vi "Main_09a refactored.vi"() -> ()   [LabVIEW 2020]
uses:
  Cluster_Point.ctl
panel:
  out "Tail Track":set{T1}(c389)
  in  "Puzzle Description":string="--- Day 9: Rope Bridge ---\nThis rope bridge creaks as you walk along it. You aren't sure how old it is, or whether it can even support your weight.\n\nIt seems to support the Elves just fine, though. The bridge spans a gorge which was carved out by the massive river far below you.\n\nYou step carefully; as you do, the ropes stretch and twist. You decide to distract yourself by modeling rope physics; maybe you can even figure out where not to step.\n\nConsider a rope with a knot at each end; these knots mark the head and the tail of the rope. If the head moves far enough away from the tail, the tail is pulled toward the head.\n\nDue to nebulous reasoning involving Planck lengths, you should be able to model the positions of the knots on a two-dimensional grid. Then, by following a hypothetical series of motions (your puzzle input) for the head, you can determine how the tail will move.\n\nDue to the aforementioned Planck lengths, the rope must be quite short; in fact, the head (H) and tail (T) must always be touching (diagonally adjacent and even overlapping both count as touching):\n\n....\n.TH.\n....\n\n....\n.H..\n..T.\n....\n\n...\n.H. (H covers T)\n...\nIf the head is ever two steps directly up, down, left, or right from the tail, the tail must also move one step in that direction so it remains close enough:\n\n.....    .....    .....\n.TH.. -> .T.H. -> ..TH.\n.....    .....    .....\n\n...    ...    ...\n.T.    .T.    ...\n.H. -> ... -> .T.\n...    .H.    .H.\n...    ...    ...\nOtherwise, if the head and tail aren't touching and aren't in the same row or column, the tail always moves one step diagonally to keep up:\n\n.....    .....    .....\n.....    ..H..    ..H..\n..H.. -> ..... -> ..T..\n.T...    .T...    .....\n.....    .....    .....\n\n.....    .....    .....\n.....    .....    .....\n..H.. -> ...H. -> ..TH.\n.T...    .T...    .....\n.....    .....    .....\nYou just need to work out where the tail goes as the head follows a series of motions. Assume the head and the tail both start at the same position, overlapping.\n\nFor example:\n\nR 4\nU 4\nL 3\nD 1\nR 4\nD 1\nL 5\nR 2\nThis series of motions moves the head right four steps, then up four steps, then left three steps, then down one step, and so on. After each step, you'll need to update the position of the tail if the step means the head is no longer adjacent to the tail. Visually, these motions occur as follows (s marks the starting position as a reference point):\n\n== Initial State ==\n\n......\n......\n......\n......\nH.....  (H covers T, s)\n\n== R 4 ==\n\n......\n......\n......\n......\nTH....  (T covers s)\n\n......\n......\n......\n......\nsTH...\n\n......\n......\n......\n......\ns.TH..\n\n......\n......\n......\n......\ns..TH.\n\n== U 4 ==\n\n......\n......\n......\n....H.\ns..T..\n\n......\n......\n....H.\n....T.\ns.....\n\n......\n....H.\n....T.\n......\ns.....\n\n....H.\n....T.\n......\n......\ns.....\n\n== L 3 ==\n\n...H..\n....T.\n......\n......\ns.....\n\n..HT..\n......\n......\n......\ns.....\n\n.HT...\n......\n......\n......\ns.....\n\n== D 1 ==\n\n..T...\n.H....\n......\n......\ns.....\n\n== R 4 ==\n\n..T...\n..H...\n......\n......\ns.....\n\n..T...\n...H..\n......\n......\ns.....\n\n......\n...TH.\n......\n......\ns.....\n\n......\n....TH\n......\n......\ns.....\n\n== D 1 ==\n\n......\n....T.\n.....H\n......\ns.....\n\n== L 5 ==\n\n......\n....T.\n....H.\n......\ns.....\n\n......\n....T.\n...H..\n......\ns.....\n\n......\n......\n..HT..\n......\ns.....\n\n......\n......\n.HT...\n......\ns.....\n\n......\n......\nHT....\n......\ns.....\n\n== R 2 ==\n\n......\n......\n.H....  (H covers T)\n......\ns.....\n\n......\n......\n.TH...\n......\ns.....\nAfter simulating the rope, you can count up all of the positions the tail visited at least once. In this diagram, s again marks the starting position (which the tail also visited) and # marks other positions the tail visited:\n\n..##..\n...##.\n.####.\n....#.\ns###..\nSo, there are 13 positions the tail visited at least once.\n\nSimulate your complete hypothetical series of motions. How many positions does the tail of the rope visit at least once?"
  out "Tail Positon count":i32
  in  "Puzzle":string="R 1\nD 1\nL 1\nD 1\nR 2\nL 1\nU 2\nD 1\nU 2\nL 1\nU 1\nL 2\nD 1\nU 2\nL 1\nR 1\nD 1\nL 2\nD 2\nL 2\nR 1\nL 2\nU 2\nR 2\nL 2\nU 2\nL 1\nD 1\nL 2\nU 1\nR 1\nD 2\nL 2\nU 1\nR 1\nD 1\nU 2\nL 1\nD 2\nU 1\nD 1\nR 2\nD 1\nL 2\nD 1\nL 1\nR 1\nD 2\nL 1\nR 2\nD 2\nU 2\nR 2\nD 2\nR 2\nL 2\nD 2\nL 2\nD 1\nU 2\nR 1\nD 2\nL 2\nR 2\nL 1\nD 1\nU 2\nD 1\nR 2\nU 2\nR 2\nD 1\nL 1\nU 2\nD 1\nU 1\nD 2\nU 1\nR 1\nU 2\nD 1\nL 2\nU 1\nL 2\nD 2\nR 1\nU 2\nL 1\nD 2\nR 1\nU 1\nD 1\nL 2\nU 1\nR 1\nD 2\nU 2\nL 1\nU 2\nD 2\nR 1\nU 2\nR 1\nU 2\nR 1\nD 2\nU 1\nD 2\nL 2\nD 2\nL 2\nD 2\nR 1\nU 1\nD 3\nU 1\nR 2\nU 3\nD 1\nU 2\nD 2\nU 2\nD 1\nU 2\nR 2\nL 2\nU 1\nL 3\nD 1\nR 3\nD 3\nR 2\nL 1\nU 3\nD 1\nU 2\nR 2\nD 1\nR 3\nD 2\nR 3\nD 1\nU 3\nL 3\nR 2\nU 3\nL 3\nU 2\nL 3\nD 1\nR 3\nU 3\nR 2\nD 1\nU 3\nR 3\nD 1\nL 2\nD 2\nL 2\nD 3\nR 2\nU 3\nL 3\nD 2\nU 3\nL 2\nU 3\nD 1\nL 1\nD 3\nR 1\nD 3\nU 1\nL 3\nU 1\nD 2\nU 1\nD 1\nU 2\nD 3\nL 1\nU 1\nR 1\nU 3\nD 3\nR 1\nL 2\nR 3\nL 3\nU 1\nD 2\nR 2\nU 2\nD 3\nU 2\nD 3\nL 1\nR 3\nD 3\nR 2\nU 3\nD 3\nL 2\nR 3\nD 3\nR 2\nL 1\nR 3\nD 2\nR 1\nD 3\nL 1\nU 1\nD 2\nR 1\nD 1\nL 1\nR 2\nL 1\nU 1\nL 2\nD 2\nL 2\nD 1\nL 2\nU 3\nD 1\nR 3\nL 2\nR 1\nL 2\nR 3\nU 2\nL 4\nR 3\nL 1\nR 2\nD 2\nL 4\nU 3\nL 1\nD 1\nL 3\nU 2\nL 3\nU 2\nL 1\nR 2\nL 3\nU 1\nD 2\nR 1\nL 4\nR 4\nL 4\nU 2\nD 2\nR 2\nL 2\nU 2\nR 1\nD 3\nL 4\nR 2\nU 1\nL 4\nR 1\nL 1\nD 4\nR 3\nD 1\nR 2\nL 2\nR 3\nL 1\nU 1\nD 3\nU 2\nR 1\nL 1\nD 3\nR 2\nU 2\nR 3\nU 2\nD 1\nR 4\nU 4\nD 3\nU 3\nR 2\nU 1\nL 1\nU 4\nD 1\nR 4\nD 4\nL 3\nU 4\nR 4\nL 1\nR 1\nU 2\nR 4\nD 2\nR 1\nU 2\nL 1\nD 1\nL 3\nR 3\nL 3\nD 3\nL 4\nD 2\nU 2\nD 3\nR 1\nU 1\nD 3\nU 1\nR 3\nD 2\nL 3\nR 2\nD 1\nL 3\nD 3\nU 3\nD 4\nL 2\nU 3\nD 5\nL 2\nD 2\nR 2\nL 3\nD 5\nU 4\nR 1\nD 5\nR 1\nD 1\nL 2\nR 4\nU 2\nD 3\nR 5\nL 2\nR 2\nD 1\nR 2\nU 5\nL 4\nU 5\nD 1\nL 2\nU 2\nR 2\nD 4\nU 3\nL 2\nD 1\nU 4\nL 4\nD 3\nL 3\nD 3\nR 1\nU 1\nR 1\nU 1\nR 2\nD 3\nR 5\nU 1\nD 2\nL 5\nU 5\nL 4\nD 4\nU 4\nL 1\nR 5\nU 2\nL 3\nU 2\nD 3\nL 5\nD 5\nL 2\nU 2\nD 4\nU 3\nD 3\nL 1\nD 2\nR 2\nD 1\nR 4\nL 3\nD 1\nU 4\nL 1\nR 2\nL 4\nD 5\nR 3\nD 1\nL 5\nD 5\nU 3\nR 2\nD 4\nL 2\nR 2\nD 3\nR 3\nU 2\nR 5\nU 4\nR 3\nL 1\nD 2\nU 1\nL 1\nR 2\nU 4\nD 4\nL 1\nR 1\nU 4\nL 3\nU 5\nR 3\nL 4\nD 3\nU 1\nR 4\nU 1\nL 1\nU 3\nR 4\nL 5\nD 1\nU 4\nR 5\nL 1\nR 4\nD 2\nL 6\nD 5\nU 5\nL 5\nR 6\nD 1\nU 2\nR 1\nU 4\nD 6\nL 6\nD 6\nU 6\nD 4\nU 4\nD 1\nU 3\nL 5\nD 6\nR 1\nL 1\nD 2\nL 4\nD 4\nL 4\nR 4\nU 2\nL 3\nD 4\nR 3\nD 4\nU 5\nR 4\nU 1\nR 6\nL 3\nR 2\nU 1\nL 1\nR 2\nD 3\nR 6\nD 6\nU 1\nD 3\nU 4\nD 5\nL 5\nU 3\nD 6\nL 5\nR 5\nU 1\nR 4\nD 2\nL 2\nR 4\nL 5\nR 4\nL 3\nD 5\nR 6\nL 6\nU 1\nR 5\nU 6\nD 2\nR 2\nD 1\nL 6\nU 4\nL 1\nR 5\nL 1\nR 2\nD 1\nL 4\nU 4\nL 1\nR 3\nU 5\nL 2\nD 6\nU 5\nR 6\nD 6\nU 3\nL 3\nU 3\nL 4\nD 5\nU 2\nD 4\nU 5\nR 6\nU 5\nD 2\nU 6\nD 3\nL 3\nD 6\nL 5\nR 2\nD 6\nR 7\nD 3\nL 7\nD 3\nU 2\nR 7\nU 2\nL 6\nR 7\nD 3\nR 7\nU 5\nR 7\nL 5\nR 7\nL 7\nU 4\nD 4\nU 1\nD 3\nU 1\nD 5\nR 3\nU 1\nD 2\nU 1\nL 4\nU 2\nL 6\nD 7\nU 1\nD 4\nU 6\nL 4\nR 4\nD 4\nR 6\nD 7\nR 1\nD 7\nL 4\nR 4\nL 1\nU 1\nR 6\nL 7\nD 7\nL 5\nU 7\nD 3\nL 6\nD 6\nU 4\nR 1\nL 2\nD 4\nR 3\nL 1\nR 7\nD 1\nL 2\nU 1\nD 2\nR 1\nU 3\nD 4\nL 3\nU 6\nL 4\nR 2\nL 1\nU 6\nD 1\nR 5\nU 2\nD 2\nL 7\nU 2\nR 5\nD 2\nR 4\nD 4\nR 3\nL 2\nR 3\nU 7\nL 5\nR 7\nU 2\nL 7\nD 3\nU 6\nD 4\nU 4\nD 6\nU 3\nL 6\nR 4\nD 2\nR 4\nD 2\nR 3\nL 5\nD 1\nU 7\nD 4\nL 4\nU 2\nD 2\nU 7\nL 5\nR 6\nU 8\nL 7\nD 2\nU 1\nR 6\nD 4\nL 4\nR 7\nD 1\nL 6\nD 7\nR 7\nU 3\nL 6\nU 1\nL 8\nD 6\nU 8\nL 7\nU 5\nD 8\nL 2\nD 3\nL 8\nU 1\nD 5\nL 4\nR 6\nD 8\nL 6\nU 5\nR 3\nU 7\nR 6\nU 3\nL 3\nD 4\nR 4\nL 2\nR 6\nD 3\nR 3\nL 8\nU 2\nD 6\nU 3\nD 8\nU 6\nD 4\nU 8\nR 7\nD 2\nU 6\nD 6\nR 1\nU 3\nD 3\nR 1\nU 3\nR 1\nD 7\nL 8\nR 8\nU 7\nR 3\nL 8\nU 2\nL 8\nD 4\nU 4\nR 1\nD 3\nR 4\nU 3\nL 7\nU 2\nR 7\nD 2\nU 4\nD 3\nL 8\nD 5\nL 3\nU 4\nD 6\nL 5\nD 2\nU 1\nR 6\nL 4\nR 6\nU 5\nR 8\nU 8\nD 7\nL 5\nD 2\nL 8\nU 2\nD 1\nR 1\nL 7\nU 4\nR 2\nU 7\nD 6\nR 6\nL 5\nU 8\nD 7\nR 8\nL 8\nD 6\nU 6\nR 1\nD 5\nL 7\nR 8\nL 4\nD 3\nL 2\nU 5\nR 9\nL 8\nD 8\nL 2\nR 4\nL 7\nR 5\nL 1\nR 8\nD 8\nL 4\nU 2\nD 7\nL 7\nD 6\nR 8\nL 3\nD 7\nU 1\nR 6\nD 6\nU 6\nL 9\nD 1\nR 7\nL 5\nR 5\nU 5\nD 4\nL 8\nU 4\nD 8\nR 4\nD 6\nU 3\nD 7\nL 5\nD 6\nR 9\nU 4\nR 6\nL 3\nU 4\nD 9\nL 7\nR 5\nD 9\nL 6\nU 7\nL 7\nR 4\nD 5\nR 7\nL 5\nR 3\nU 8\nL 6\nU 5\nL 9\nR 8\nU 4\nD 2\nL 4\nD 7\nR 7\nD 4\nL 4\nU 2\nL 3\nR 1\nD 3\nU 6\nR 1\nU 8\nR 2\nL 4\nD 3\nL 5\nU 4\nR 7\nL 2\nR 7\nL 9\nD 9\nU 5\nL 4\nU 1\nD 1\nU 6\nD 1\nL 6\nD 7\nU 5\nD 9\nR 9\nD 5\nU 9\nL 3\nR 5\nD 10\nR 1\nU 7\nD 6\nL 3\nU 5\nR 1\nD 5\nR 8\nU 3\nL 1\nD 2\nR 1\nL 6\nR 8\nD 9\nU 9\nD 4\nR 1\nU 8\nL 5\nU 4\nD 7\nL 1\nR 4\nL 6\nD 4\nR 5\nD 1\nR 10\nD 5\nR 7\nU 6\nR 5\nU 2\nL 8\nR 1\nU 3\nL 5\nU 4\nL 3\nD 3\nU 6\nD 10\nL 3\nD 7\nL 5\nD 4\nU 6\nR 9\nU 5\nD 5\nR 2\nL 7\nU 8\nD 5\nR 9\nL 6\nR 8\nU 9\nL 4\nR 10\nD 10\nL 9\nR 8\nL 4\nR 5\nL 9\nD 1\nL 3\nR 9\nU 2\nL 5\nR 2\nU 1\nR 4\nD 10\nU 3\nD 8\nL 9\nD 8\nL 5\nD 4\nU 2\nL 8\nR 5\nU 4\nD 1\nL 4\nU 7\nD 9\nR 3\nD 7\nR 9\nL 6\nR 6\nU 8\nL 10\nU 5\nD 4\nR 5\nL 6\nD 7\nL 10\nR 1\nL 9\nU 6\nD 9\nR 7\nL 7\nD 6\nU 6\nR 1\nD 7\nL 1\nR 9\nD 9\nR 3\nL 5\nD 4\nR 3\nL 5\nD 11\nU 1\nR 6\nD 8\nR 4\nD 3\nR 9\nU 3\nD 8\nU 7\nR 2\nU 10\nR 4\nL 4\nD 10\nR 8\nU 11\nR 7\nD 7\nR 9\nD 11\nU 6\nR 7\nD 10\nL 4\nD 5\nL 7\nD 3\nL 4\nD 4\nU 4\nR 3\nL 9\nD 4\nL 8\nU 5\nR 7\nL 2\nD 4\nR 11\nU 10\nD 3\nR 8\nD 3\nR 10\nL 8\nU 6\nR 4\nD 10\nR 7\nD 3\nR 2\nU 1\nD 5\nL 8\nU 2\nR 1\nU 8\nR 11\nL 3\nU 10\nL 5\nD 3\nL 6\nU 10\nL 11\nD 4\nL 5\nD 1\nL 4\nD 1\nL 3\nR 7\nU 7\nR 4\nL 1\nU 10\nD 11\nL 1\nR 1\nU 9\nD 6\nL 9\nD 1\nL 4\nD 11\nL 5\nU 2\nL 5\nD 8\nU 10\nD 5\nU 10\nL 8\nR 11\nD 10\nU 11\nR 4\nU 6\nD 11\nR 1\nL 4\nU 12\nL 8\nU 12\nD 4\nL 7\nU 7\nL 8\nD 3\nU 1\nL 12\nD 5\nU 3\nD 6\nR 7\nU 1\nD 12\nR 6\nU 3\nD 3\nR 12\nU 5\nR 3\nU 8\nL 6\nR 6\nU 3\nL 4\nD 8\nL 5\nD 12\nU 1\nL 9\nR 4\nL 1\nD 6\nU 9\nL 5\nR 3\nL 9\nD 8\nR 6\nD 3\nU 6\nL 1\nD 7\nU 5\nD 1\nL 11\nR 7\nD 11\nL 3\nU 6\nR 9\nD 12\nR 11\nL 5\nR 8\nL 2\nU 10\nR 6\nU 10\nL 9\nU 1\nL 1\nR 8\nL 7\nR 3\nU 4\nL 3\nR 8\nL 9\nR 11\nL 9\nD 11\nU 1\nL 12\nR 6\nL 3\nR 3\nD 12\nU 9\nL 9\nD 8\nR 4\nL 7\nR 1\nU 2\nR 4\nU 4\nR 11\nU 7\nD 11\nU 3\nD 6\nU 7\nL 2\nD 4\nU 9\nR 3\nL 8\nR 9\nL 4\nR 5\nL 7\nD 3\nR 8\nL 6\nU 10\nR 3\nL 6\nD 8\nU 3\nD 9\nL 1\nU 13\nR 12\nL 13\nR 2\nU 8\nR 1\nD 11\nR 5\nL 4\nU 5\nL 3\nD 13\nU 2\nD 1\nU 2\nL 9\nD 3\nR 6\nU 13\nL 3\nU 5\nR 2\nD 2\nL 5\nU 4\nR 6\nD 1\nU 9\nL 7\nR 11\nU 10\nD 12\nR 10\nU 7\nR 5\nL 2\nR 13\nL 13\nD 3\nR 7\nU 1\nL 1\nD 2\nL 9\nU 12\nD 7\nU 13\nL 12\nU 13\nD 7\nU 7\nD 8\nL 2\nU 6\nD 2\nU 6\nL 8\nU 4\nD 11\nU 11\nL 11\nR 10\nL 10\nR 6\nD 13\nU 2\nL 7\nU 8\nD 1\nR 6\nL 7\nR 9\nL 8\nR 9\nL 6\nR 7\nD 12\nR 11\nL 8\nR 1\nD 5\nR 5\nL 10\nU 6\nL 8\nD 9\nL 5\nU 4\nD 12\nU 8\nL 13\nU 6\nD 10\nR 5\nL 13\nD 7\nL 13\nR 5\nL 10\nD 13\nL 9\nR 3\nD 8\nU 9\nD 10\nU 10\nD 7\nL 5\nR 5\nD 9\nL 7\nR 10\nD 13\nR 1\nU 2\nR 6\nU 14\nR 10\nD 6\nU 13\nD 14\nU 5\nD 1\nU 8\nR 4\nU 9\nR 13\nL 4\nD 2\nR 8\nU 2\nD 12\nU 3\nR 6\nU 6\nD 11\nR 7\nL 12\nR 9\nU 7\nD 1\nR 14\nL 11\nU 4\nD 13\nU 5\nL 7\nR 14\nL 1\nU 6\nD 3\nL 1\nU 13\nD 8\nU 14\nD 5\nU 14\nL 1\nR 1\nD 5\nU 7\nL 8\nR 6\nU 1\nD 2\nR 14\nU 13\nL 10\nU 8\nD 13\nU 6\nR 2\nD 4\nR 6\nU 7\nD 10\nL 6\nU 5\nL 3\nD 9\nU 13\nD 8\nU 3\nR 3\nL 12\nD 5\nR 8\nU 7\nR 11\nU 6\nD 7\nR 13\nU 1\nD 9\nU 10\nD 3\nL 5\nR 12\nL 4\nD 13\nR 7\nD 12\nR 11\nD 9\nR 5\nU 13\nR 3\nD 4\nU 10\nR 3\nU 6\nL 4\nR 1\nU 4\nL 9\nD 11\nU 5\nD 3\nU 13\nD 1\nL 1\nD 13\nL 2\nR 9\nL 4\nR 2\nU 9\nD 9\nU 12\nL 14\nR 2\nL 9\nR 5\nU 2\nD 3\nR 13\nU 5\nD 1\nU 15\nR 6\nD 14\nR 8\nL 9\nD 14\nL 6\nR 8\nU 14\nR 11\nL 3\nD 15\nU 5\nR 1\nL 7\nR 12\nD 1\nR 4\nD 13\nU 9\nD 2\nL 3\nU 10\nR 10\nD 2\nR 6\nU 13\nD 7\nR 5\nU 5\nL 12\nU 6\nR 1\nL 7\nU 9\nD 15\nL 8\nU 9\nL 5\nR 3\nL 9\nU 6\nL 11\nD 8\nL 11\nD 13\nU 3\nR 6\nD 2\nL 10\nR 15\nU 2\nD 8\nR 6\nD 6\nL 8\nD 7\nU 2\nD 14\nU 4\nR 6\nD 15\nL 12\nR 4\nD 3\nU 7\nD 10\nL 8\nU 7\nR 10\nU 11\nD 2\nR 10\nD 10\nU 13\nR 8\nL 2\nU 12\nR 9\nU 12\nR 5\nU 10\nL 6\nR 3\nD 10\nL 10\nU 6\nL 4\nR 3\nD 9\nR 15\nD 14\nL 11\nR 5\nU 2\nR 14\nL 15\nR 3\nD 3\nL 4\nU 10\nD 14\nL 9\nD 5\nL 16\nU 12\nL 4\nD 15\nL 10\nR 14\nD 4\nR 12\nL 7\nU 5\nR 3\nL 6\nU 16\nL 5\nU 8\nD 8\nL 6\nD 3\nU 14\nR 1\nL 13\nU 4\nD 11\nR 5\nL 11\nD 7\nR 1\nL 14\nU 10\nL 5\nD 15\nU 14\nL 4\nD 7\nU 3\nR 1\nU 2\nR 3\nD 16\nU 7\nR 7\nD 13\nR 7\nD 5\nU 7\nR 16\nU 4\nL 3\nR 9\nU 1\nD 2\nR 5\nD 3\nU 8\nR 5\nL 13\nU 13\nL 2\nR 9\nL 14\nD 10\nR 1\nU 1\nR 14\nU 14\nR 2\nL 1\nR 12\nL 1\nD 6\nR 2\nD 7\nR 11\nL 5\nD 8\nR 15\nD 12\nR 12\nL 8\nD 10\nR 2\nD 12\nU 15\nL 9\nD 4\nU 3\nL 8\nD 3\nU 9\nD 16\nL 2\nU 14\nR 15\nD 14\nU 12\nD 6\nU 14\nR 11\nD 12\nR 2\nU 13\nL 2\nR 1\nD 6\nU 13\nD 15\nU 1\nR 14\nL 16\nD 8\nR 13\nL 14\nR 3\nD 8\nL 6\nR 16\nD 6\nL 13\nR 2\nL 11\nD 2\nU 1\nR 15\nL 9\nU 1\nR 12\nL 9\nD 7\nL 8\nU 2\nL 14\nR 7\nU 8\nD 15\nR 8\nD 13\nL 15\nR 11\nD 17\nU 2\nR 14\nL 9\nU 11\nD 6\nU 4\nD 8\nU 16\nD 5\nL 3\nD 11\nL 7\nU 11\nL 4\nD 5\nL 5\nD 2\nU 8\nR 17\nD 17\nU 12\nR 4\nL 13\nR 15\nL 10\nU 2\nL 10\nR 6\nD 1\nU 6\nL 3\nD 8\nR 4\nD 1\nL 4\nD 13\nR 1\nU 3\nL 1\nU 9\nD 13\nU 2\nD 13\nR 6\nD 8\nR 6\nD 13\nR 4\nD 10\nL 10\nU 8\nD 1\nR 6\nU 14\nR 3\nL 10\nU 15\nL 11\nU 13\nL 4\nU 5\nL 16\nR 16\nU 11\nR 14\nD 7\nU 5\nR 9\nL 5\nU 12\nR 16\nU 10\nD 5\nR 17\nL 3\nD 5\nU 13\nR 3\nU 3\nL 14\nU 1\nL 8\nR 2\nD 3\nU 9\nD 7\nL 1\nD 5\nR 16\nD 12\nR 1\nU 2\nL 16\nU 3\nR 18\nD 11\nR 3\nL 17\nR 7\nL 6\nD 13\nL 5\nR 12\nD 3\nU 1\nL 1\nU 5\nL 8\nR 11\nL 13\nD 14\nR 17\nD 17\nL 2\nU 7\nD 18\nR 3\nD 2\nU 6\nD 9\nR 3\nU 3\nR 5\nD 16\nR 9\nD 13\nU 8\nD 17\nR 4\nL 6\nR 7\nD 2\nR 15\nU 10\nR 15\nD 6\nL 8\nR 17\nD 5\nL 9\nU 18\nD 10\nU 3\nL 6\nU 10\nD 10\nU 16\nR 6\nD 18\nU 10\nD 8\nU 14\nR 3\nU 14\nL 16\nR 3\nD 5\nL 2\nR 4\nD 9\nL 13\nR 17\nL 8\nD 2\nR 16\nD 18\nL 11\nD 15\nU 5\nD 7\nU 14\nD 13\nU 7\nL 13\nD 13\nR 1\nD 15\nR 11\nL 1\nU 6\nD 14\nL 6\nU 8\nD 15\nR 8\nL 12\nD 17\nR 8\nL 17\nD 16\nR 9\nD 19\nU 4\nR 9\nU 10\nL 3\nU 3\nD 5\nR 2\nU 6\nL 16\nD 8\nR 4\nL 16\nR 15\nU 6\nL 8\nD 6\nL 6\nR 1\nL 8\nD 13\nL 1\nU 7\nR 16\nL 16\nU 1\nL 18\nD 16\nL 8\nU 2\nD 1\nR 2\nD 10\nU 8\nD 2\nR 18\nU 14\nD 15\nR 15\nU 3\nD 1\nU 17\nL 17\nD 15\nL 14\nR 6\nL 18\nU 19\nL 6\nU 17\nL 1\nD 2\nU 17\nR 11\nL 3\nR 3\nL 12\nU 1\nL 9\nU 13\nD 15\nU 12\nR 1\nL 5\nD 17\nL 14\nD 13\nL 2\nD 10\nU 5\nR 13\nL 19\nD 1\nR 12\nU 17\nR 15\nD 19\nU 12\nD 16\nR 2\nU 3\nR 15\nL 13\nU 11\nD 19\nR 10\nD 19\nL 2\nU 12\nR 5\nL 13\nU 13\nR 1\nD 11\nR 17\nD 7\nU 4\nD 14\nL 13\nR 8\nL 8\nD 8"
  in  "Example":string="R 4\nU 4\nL 3\nD 1\nR 4\nD 1\nL 5\nR 2"
  # "5874"
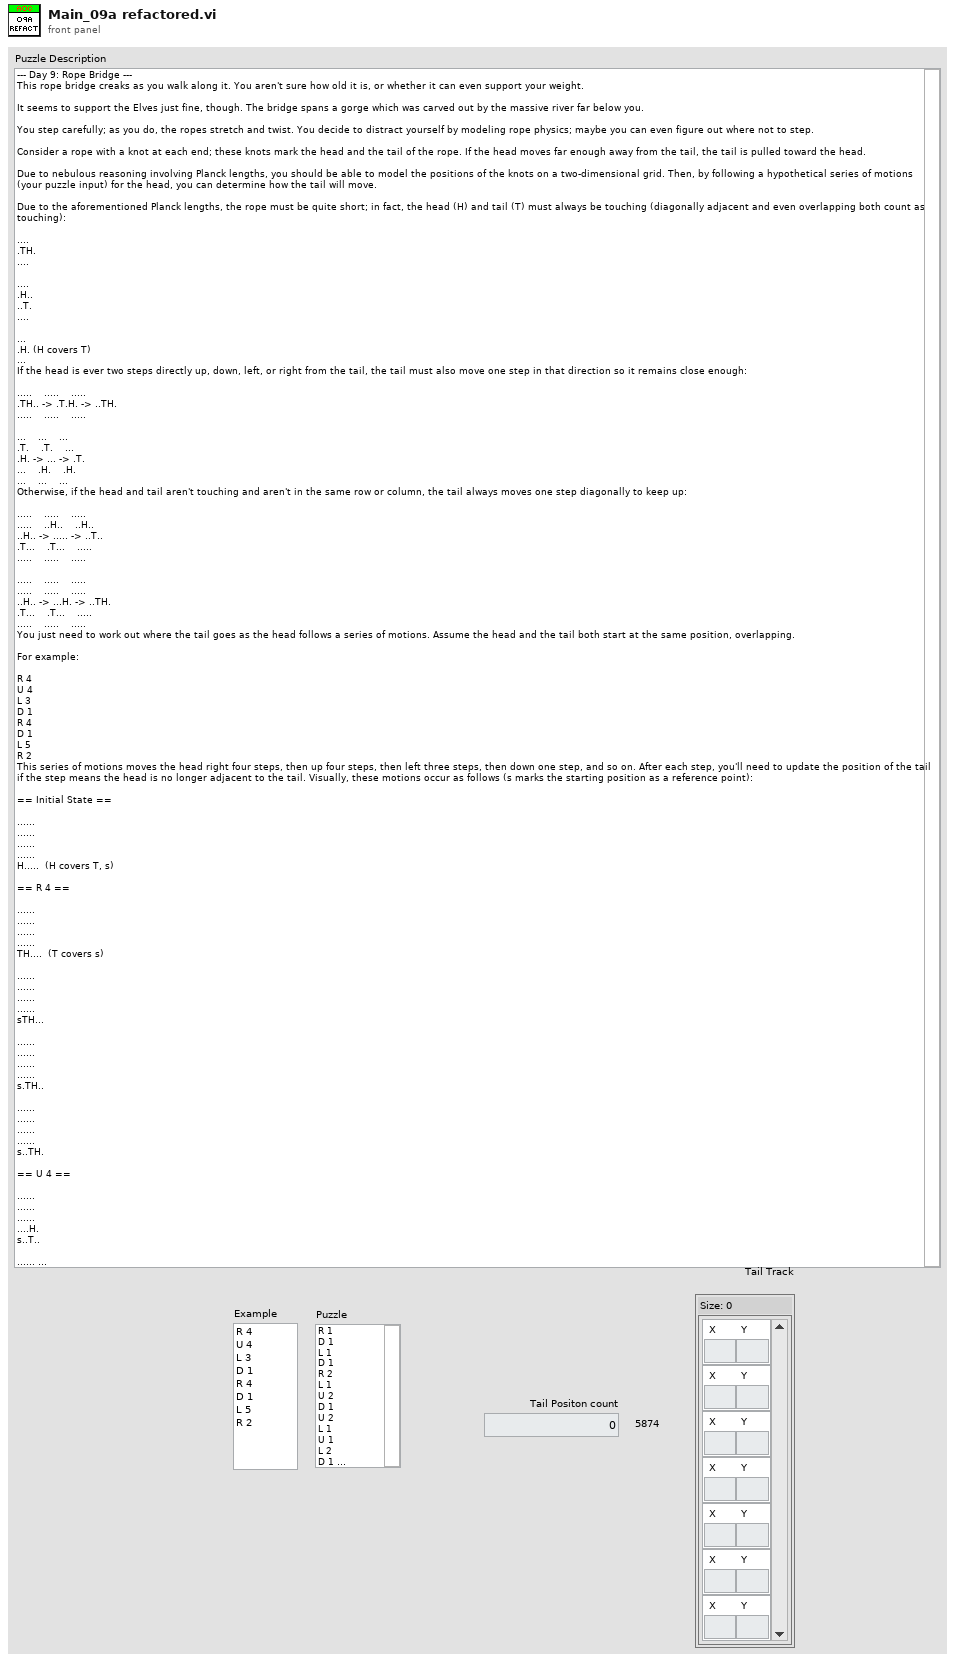
[diagram p1: front panel]
types:
  T1 = typedef "Cluster_Point.ctl" = cluster{"X":i32, "Y":i32}
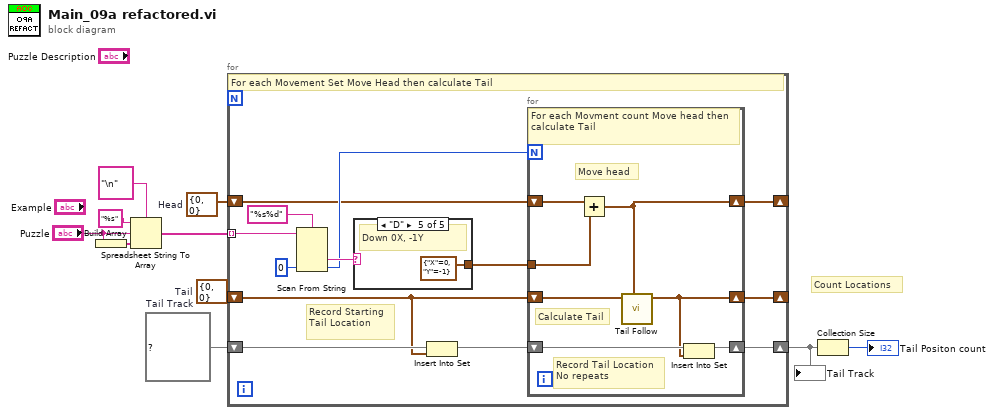
[diagram p0: block diagram]
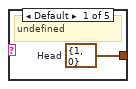
[diagram p2: hidden frame]
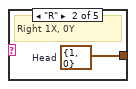
[diagram p3: hidden frame]
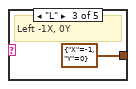
[diagram p4: hidden frame]
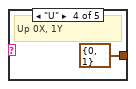
[diagram p5: hidden frame]
diagram:
  w6 = set{T1} {}  # Tail Track
  w5 = T1 {"X"=0, "Y"=0}  # Tail
  w4 = T1 {"X"=0, "Y"=0}  # Head
  # "Count Locations"
  n1 = Build Array("Puzzle") -> (w10:string[])
  n2 = Spreadsheet String To Array(delimiter (Tab)="\n", format string="%s", spreadsheet string="Puzzle", array type (2D Dbl)=w10) -> (array=w7:string[])
  n3 = for {
    tunnel: w7 -> [w22] mode=indexing
    shift-right: [w17] -> _
    shift-left: w4 -> [w18]
    shift-right: [w16] -> _
    shift-left: w5 -> [w11]
    shift-right: [w15] -> w3
    shift-left: w6 -> [w13]
    # "Record Starting \nTail Location"
    # "For each Movement Set Move Head then calculate Tail"
    n4 = Scan From String(format string="%s%d", input string=w22, default 2=0 ("default value 2")) -> (output 1=w21:string, output 2=w19:i32)  [unwired: 3 in, 3 out]
    n5 = case shown="\"D\"" w21 {
      tunnel: [w31 w32 T1 {"X"=-1, "Y"=0} ("Head") T1 {"X"=0, "Y"=1} ("Head") T1 {"X"=0, "Y"=-1} ("Head")] -> w14
      frame Default {
        w31 = T1 {"X"=1, "Y"=0}  # Head
        # "undefined"
      }
      frame "R" {
        w32 = T1 {"X"=1, "Y"=0}  # Head
        # "Right 1X, 0Y"
      }
      frame "L" {
        # "Left -1X, 0Y"
      }
      frame "U" {
        # "Up 0X, 1Y"
      }
      frame "D" {
        # "Down 0X, -1Y"
      }
    }
    n6 = Insert Into Set(10:w11, 11:w13) -> (3:w12:set{T1})  [unwired: 1 out]
    n7 = for {
      N: w19 -> [_]
      shift-right: [w25] -> w17
      shift-left: w18 -> [w30]
      shift-right: [w26] -> w16
      shift-left: w11 -> [w24]
      shift-right: [w27] -> w15
      shift-left: w12 -> [w28]
      tunnel: w14 -> [w29]
      # "Record Tail Location\nNo repeats"
      # "Calculate Tail"
      # "Move head"
      # "For each Movment count Move head then calculate Tail"
      n8 = Add(x=w30, y=w29) -> (x+y=w25:T1)
      n9 = call "Tail Follow.vi"("Head"=w25, "Tail"=w24) -> ("Tail Out"=w26:T1)  [unwired: 9 in]
      n10 = Insert Into Set(10:w26, 11:w28) -> (3:w27:set{T1})  [unwired: 1 out]
    }
  }
  "Tail Track" <- w3
  n11 = Collection Size(1:w3) -> (0:→"Tail Positon count":i32)
